vi "Auto Shoot.vi"(4 "RPM Override?":i32, 6 "Angle Override?":i32, 8 "Angle":dbl, 9 "Right RPM":dbl, 10 "Left RPM":dbl, 11 "Shot Type":i32) -> (3 "Finished?":bool)   [LabVIEW 2015]
uses:
  Common Code/Shooter Commands.ctl
  Common Code/Shoot Modes Enum.ctl
  Common Code/Shot Type.ctl
  Common Code/Change Detect Boolean.vi
  Robot Global Data.vi
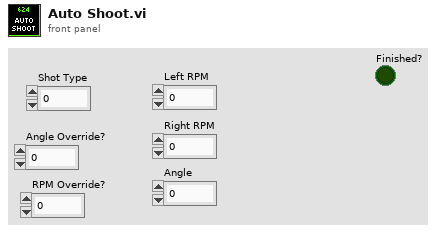
[diagram p1: front panel]
types:
  T1 = typedef "Shooter Commands.ctl" = enum16{"Idle", "Prime Shooter", "Shoot"}
  T2 = typedef "Shoot Modes Enum.ctl" = enum16{"Manual", "Safe", "Auto"}
  T3 = typedef "Shot Type.ctl" = enum16{"Batter Shot", "Corner Shot", "Curve Shot", "Vision Shot", "Deep Middle Shot"}
  T4 = typedef "Manual Shoot.ctl" = cluster{"Spin Wheels":bool, "Fire":bool, "Angle":dbl, "Angle Power":dbl, "Use Manual Angle":bool, "Override RPM":bool, "Left RPM":dbl, "Right RPM":dbl, "Secure Ball?":bool}
  T5 = typedef "Shooter State Cluster.ctl" = cluster{"State":T6, "Left RPM":dbl, "Right RPM":dbl, "Shooter Ready?":bool, "Ball Loaded?":bool, "Current Angle":dbl, "Angle Motor Output":dbl, "Trigger Output":dbl, "Angle Ready?":bool, "RPM Ready?":bool, "Vision Ready?":bool, "Ball Loaded?":bool, "Mode":T2, "Shot Type":T3, "Pot Height":dbl, "Current Tripped Forward?":bool, "Current Tripped Backward?":bool, "Left Motor":dbl, "Right Motor":dbl, "Intake High?":bool, "Raw Left Pos":dbl, "Raw Right Pos":dbl, "Raw Left V":dbl, "Raw Right V":dbl, "Right Servo":i32, "Left Servo":i32}
  T6 = typedef "Shooter State.ctl" = enum16{"Idle", "Warmup", "Shooter Ready", "Shoot"}
  T7 = typedef "Shooter Command Cluster.ctl" = cluster{"Command":T1, "Mode":T2, "Shot Type":T3, "Override Trigger IR":bool, "Override Angle?":bool}
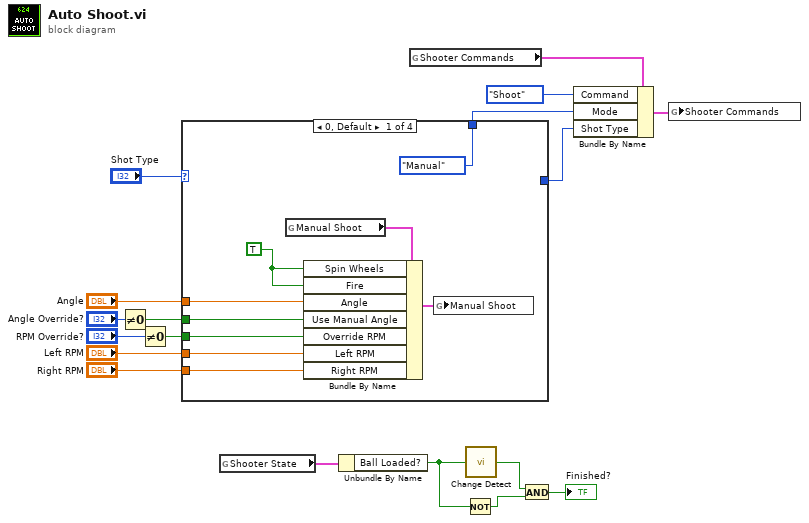
[diagram p0: block diagram]
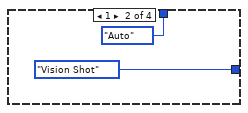
[diagram p2: hidden frame]
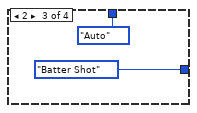
[diagram p3: hidden frame]
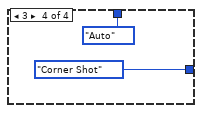
[diagram p4: hidden frame]
diagram:
  n1 = Not Equal To 0?(x="Angle Override?") -> (x != 0?=w9:bool)
  n2 = Not Equal To 0?(x="RPM Override?") -> (x != 0?=w11:bool)
  n3 = case shown="0, Default" "Shot Type" {
    tunnel: [Shoot_Modes_Enum."Manual" ("Mode") Shoot_Modes_Enum."Auto" ("Mode") Shoot_Modes_Enum."Auto" ("Mode") Shoot_Modes_Enum."Auto" ("Mode")] -> w15
    tunnel: [_ Shot_Type."Vision Shot" ("Shot Type") Shot_Type."Batter Shot" ("Shot Type") Shot_Type."Corner Shot" ("Shot Type")] -> w14
    tunnel: w11 -> [w23 _ _ _]
    tunnel: w9 -> [w22 _ _ _]
    tunnel: "Left RPM" -> [w21 _ _ _]
    tunnel: "Right RPM" -> [w20 _ _ _]
    tunnel: "Angle" -> [w19 _ _ _]
    frame 0, Default {
      w25 = TRUE ("Spin Wheels")
      n4 = global read "Robot Global Data.vi" "Manual Shoot"() -> (w27:T4)
      n5 = Bundle By Name(cluster=w27, "Spin Wheels"=w25, "Fire"=w25, "Angle"=w19, "Use Manual Angle"=w22, "Override RPM"=w23, "Left RPM"=w21, "Right RPM"=w20) -> (w24:T4)
      n6 = global write "Robot Global Data.vi" "Manual Shoot"(w24) -> ()
    }
    frame 1 {
    }
    frame 2 {
    }
    frame 3 {
    }
  }
  n7 = global read "Robot Global Data.vi" "Shooter State"() -> (w5:T5)
  n8 = Unbundle By Name(w5) -> ("Ball Loaded?"=w4:bool)
  n9 = global read "Robot Global Data.vi" "Shooter Commands"() -> (w18:T7)
  n10 = Not(x=w4) -> (.not. x?=w3:bool)
  n11 = call-poly "Change Detect.vi"("In"=w4) -> ("Changed?"=w2:bool)
  n12 = And(x=w2, y=w3) -> (x .and. y?=→"Finished?":bool)
  n13 = Bundle By Name(cluster=w18, "Command"=Shooter_Commands."Shoot", "Mode"=w15, "Shot Type"=w14) -> (w13:T7)
  n14 = global write "Robot Global Data.vi" "Shooter Commands"(w13) -> ()
